vi "PH_PSDBController.PC _Data Status.vi"(0 "i ref in":refnum<vi>, 2 "Data Status service name":string="N/A", 3 "Data Status":T1 items=["no info", "no Data collection", "no problem", "Error getting the ID", "Error writing Data", "Error getting the subsystem", "Error getting the Shot ID", "Error getting the Shot Types", "Error getting the Experiments", "Error verifying wanted Shottype", "Error verifying wanted Experiment"], 5 "error IO":errorcluster) -> (14 "i ref out":refnum<vi>, 19 "error out":errorcluster)   [LabVIEW 2014, in "PH_PSDBController.lvlib"]
uses:
  PH_PSDBController.lvlib
  PH_Basics/PH_PSDBWriter/PH_PSDBWriter.Data Status.ctl
  PH_Basics/PH_PSDBWriter/PH_PSDBWriter.lvlib
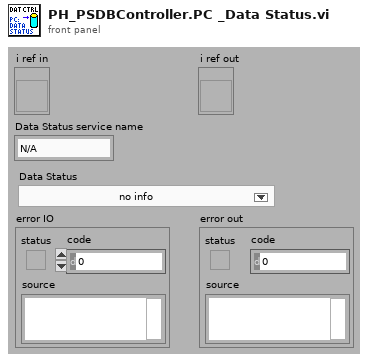
[diagram p1: front panel]
types:
  T1 = typedef "PH_PSDBWriter.lvlib/PH_PSDBWriter.Data Status.ctl" = i16
  T2 = typedef "PH_PSDBController.lvlib/PH_PSDBController.i attribute.ctl" = cluster{"GUI Refs":cluster{"Data Status":refnum<vi>, "Current Shot ID":refnum<vi>, "active Subsystems":refnum<vi>, "Experiment Description":refnum<vi>, "Shot Comment":refnum<vi>, "Experiment":refnum<vi>, "Shottype":refnum<vi>, "Sequencer SM State":refnum<vi>, "Instances with Errors":refnum<vi>}, "Service ID Shot ID":i32, "Service ID wanted Subsystem":i32, "Data Status":T1, "Shotinformation":cluster{"Current Experiment ID":i32, "Current Shot Type":i32, "Current Comment":string}, "Data taking?":bool, "Service ID current Shottype":i32, "Service ID current Experiment":i32, "Service ID currentShot Comment":i32, "Service ID possible Shottypes":i32, "Service ID possible Experiments":i32, "possible Experiments":T3[], "possible Shottypes":T3[], "List":cluster{"Info":cluster{"Instance":string, "Data Status":T1}[], "GUI Ref":refnum<vi>, "Classname":string}[], "Subsystems Off?":cluster{"PHELIX_Beamline_fs_YLF_BL_Status":bool, "PHELIX_Beamline_ns_BL_Status":bool, "PHELIX_Beamline_PA_Input_BL_Status":bool, "PHELIX_Beamline_PA_MA_BL_Status":bool, "PHELIX_Beamline_MA_Z6_BL_Status":bool, "PHELIX_Beamline_MA_LB_BL_Status":bool, "PHELIX_Beamline_PA_LL_BL_Status":bool}, "PSDB Credentials":T4}
  T3 = typedef "PSDB.lvlib/PSDB_Info.ctl" = cluster{"Name":string, "Description":string, "ID":i32}
  T4 = typedef "PH_Common.lvlib/PH_Connection.PSDB Credentials.ctl" = cluster{"PW":string, "ID":string, "DS":string}
  T5 = cluster{"Info":cluster{"Instance":string, "Data Status":T1}[], "GUI Ref":refnum<vi>, "Classname":string}[]
  T6 = cluster{"Info":cluster{"Instance":string, "Data Status":T1}[], "GUI Ref":refnum<vi>, "Classname":string}
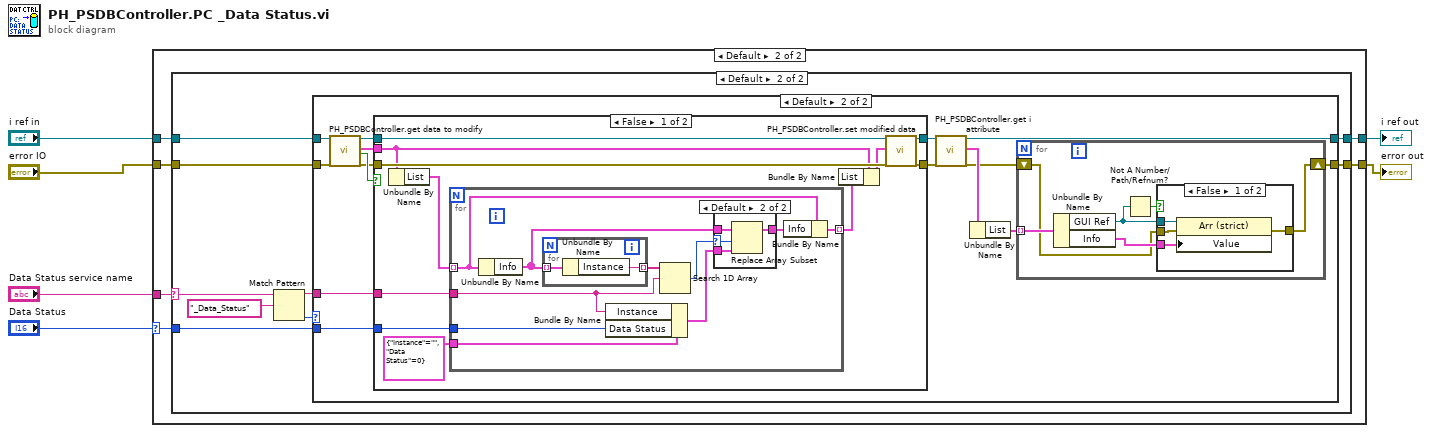
[diagram p0: block diagram]
diagram:
  n1 = case shown="Default" "Data Status" {
    selector: "Data Status" -> [_ w9]
    tunnel: [w7 w14] -> w6
    tunnel: [w8 w13] -> w5
    tunnel: "error IO" -> [w7 w12]
    tunnel: "i ref in" -> [w8 w11]
    tunnel: "Data Status service name" -> [_ w10]
    frame -1 {
    }
    frame Default {
      n2 = case shown="Default" w10 {
        selector: w10 -> [_ w19]
        tunnel: w9 -> [_ w25]
        tunnel: [w15 w24] -> w14
        tunnel: [w16 w23] -> w13
        tunnel: w12 -> [w15 w22]
        tunnel: w11 -> [w16 w21]
        frame "", "N/A" {
        }
        frame Default {
          n3 = Match Pattern(string=w19, regular expression="_Data_Status" ("string")) -> (before substring=w18:string, offset past match=w17:i32)  [unwired: 1 in, 2 out]
          n4 = case shown="Default" w17 {
            tunnel: w25 -> [_ w42]
            tunnel: [w26 w28] -> w24
            tunnel: [w27 w34] -> w23
            tunnel: w22 -> [w26 w37]
            tunnel: w21 -> [w27 w36]
            tunnel: w18 -> [_ w35]
            frame -1 {
            }
            frame Default {
              n5 = call "PH_PSDBController.get data to modify.vi"("i ref in"=w36, "error in (no error)"=w37) -> ("i ref out"=w39:refnum<vi>, "i attribute"=w41:T2, "timed out"=w40:bool, "error out"=w38:errorcluster)  [unwired: 14 in]
              n6 = case shown="False" w40 {
                tunnel: w38 -> [w62 w82]
                tunnel: w39 -> [w64 w83]
                tunnel: [w63 w83] -> w33
                tunnel: [w58 w82] -> w32
                tunnel: w41 -> [w60 _]
                tunnel: w42 -> [w56 _]
                tunnel: w35 -> [w57 _]
                frame False {
                  n7 = Unbundle By Name(w60) -> ("List"=w61:T5)
                  n8 = for {
                    tunnel: w61 -> [w67] mode=indexing
                    tunnel: w57 -> [w71]
                    tunnel: w56 -> [w72]
                    tunnel: cluster{"Instance":string, "Data Status":T1} {"Instance"="", "Data Status"=0} ("new element/subarray") -> [w69]
                    tunnel: [w66] -> w54 mode=indexing
                    n9 = Unbundle By Name(w67) -> ("Info"=w73:cluster{"Instance":string, "Data Status":T1}[])
                    n10 = for {
                      tunnel: w73 -> [w81] mode=indexing
                      tunnel: [w80] -> w74 mode=indexing
                      n11 = Unbundle By Name(w81) -> ("Instance"=w80:string)
                    }
                    n12 = Bundle By Name(cluster=w69, "Instance"=w71, "Data Status"=w72) -> (w70:cluster{"Instance":string, "Data Status":T1})
                    n13 = Search 1D Array(1D array=w74, element=w71) -> (index of element=w68:i32)  [unwired: 1 in]
                    n14 = case shown="Default" w68 {
                      selector: w68 -> [_ w76]
                      tunnel: w73 -> [w75 w79]
                      tunnel: w70 -> [_ w78]
                      tunnel: [w75 w77] -> w65
                      frame -1 {
                      }
                      frame Default {
                        n15 = Replace Array Subset(array=w79, new element=w78, index=w76) -> (w77:cluster{"Instance":string, "Data Status":T1}[])
                      }
                    }
                    n16 = Bundle By Name(cluster=w67, "Info"=w65) -> (w66:T6)
                  }
                  n17 = Bundle By Name(cluster=w60, "List"=w54) -> (w59:T2)
                  n18 = call "PH_PSDBController.set modified data.vi"("i ref in"=w64, "i attribute"=w59, "error in (no error)"=w62) -> ("i ref out"=w63:refnum<vi>, "error out"=w58:errorcluster)  [unwired: 15 in]
                }
                frame True {
                }
              }
              n19 = call "PH_PSDBController.get i attribute.vi"("i ref in"=w33, "error in (no error)"=w32) -> ("i ref out"=w34:refnum<vi>, "i attribute"=w31:T2, "error out"=w29:errorcluster)  [unwired: 15 in]
              n20 = Unbundle By Name(w31) -> ("List"=w30:T5)
              n21 = for {
                tunnel: w30 -> [w48] mode=indexing
                shift-right: [w43] -> w28
                shift-left: w29 -> [w44]
                n22 = Unbundle By Name(w48) -> ("GUI Ref"=w46:refnum<vi>, "Info"=w47:cluster{"Instance":string, "Data Status":T1}[])
                n23 = Not A Number/Path/Refnum?(number/path/refnum=w46) -> (NaN/Path/Refnum?=w45:bool)
                n24 = case shown="False" w45 {
                  tunnel: w46 -> [w52 _]
                  tunnel: w47 -> [w51 _]
                  tunnel: w44 -> [w50 w53]
                  tunnel: [w49 w53] -> w43
                  frame False {
                    n25 = property class="Arr (strict)"(reference=w52, error in=w50, "Value"=w51) -> (error out=w49:errorcluster)  [unwired: 1 out]
                  }
                  frame True {
                  }
                }
              }
            }
          }
        }
      }
    }
  }
  "error out" <- w6
  "i ref out" <- w5
